vi "Set Direction.vi"(8 "error in (no error)":errorcluster, 10 "Direction":bool, 11 "Impulse Manager in":refnum<class "Impulse Manager.lvclass">) -> (0 "error out":errorcluster, 3 "Impulse Manager out":refnum<class "Impulse Manager.lvclass">)   [LabVIEW 2016, in "Impulse Manager.lvclass"]
uses:
  Impulse Manager.lvclass
  Impulse Manager.lvclass/Impulse Manager.ctl
  Impulse Data/Impulse Data.lvclass/Impulse Data.ctl
  Impulse Data/Impulse Data.lvclass
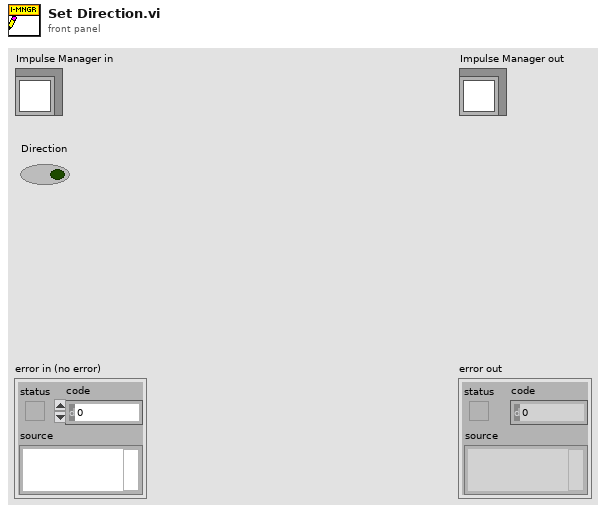
[diagram p1: front panel]
types:
  T1 = typedef "Impulse Data.lvclass/Instance handle.ctl" = refnum<data-value>
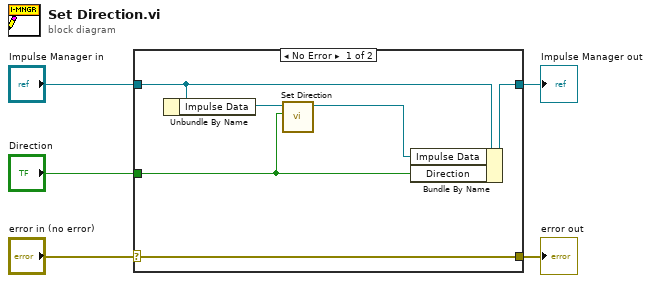
[diagram p0: block diagram]
diagram:
  n1 = case shown="No Error" "error in (no error)" {
    selector: "error in (no error)" -> [w11 w12]
    tunnel: [w11 w12] -> w4
    tunnel: [w10 w13] -> w2
    tunnel: "Impulse Manager in" -> [w9 w13]
    tunnel: "Direction" -> [w6 _]
    frame No Error {
      n2 = Unbundle By Name(w9) -> ("Impulse Data"=w8:T1)
      n3 = call "Set Direction.vi"("Direction"=w6, "Reference in"=w8) -> ("Reference out"=w7:T1)  [unwired: 9 in]
      n4 = Bundle By Name(cluster=w9, "Impulse Data"=w7, "Direction"=w6) -> (w10:refnum<class "Impulse Manager.lvclass">)
    }
    frame Error {
    }
  }
  "error out" <- w4
  "Impulse Manager out" <- w2
